vi "Generate Veristand Loopback Channels.vi"() -> (1 "Rx Aliases":string[](array[string]), 2 "Tx Aliases":string[](array[string]))   [LabVIEW 2020, in "Loopback.lvclass"]
uses:
  Loopback.lvclass
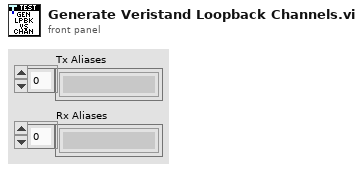
[diagram p1: front panel]
types:
  T1 = cluster{"tx terminal name":string, "rx terminal name":string, "words":i32, "parameter names":string[]}[]
  T2 = cluster{"tx terminal name":string, "rx terminal name":string, "words":i32, "parameter names":string[]}
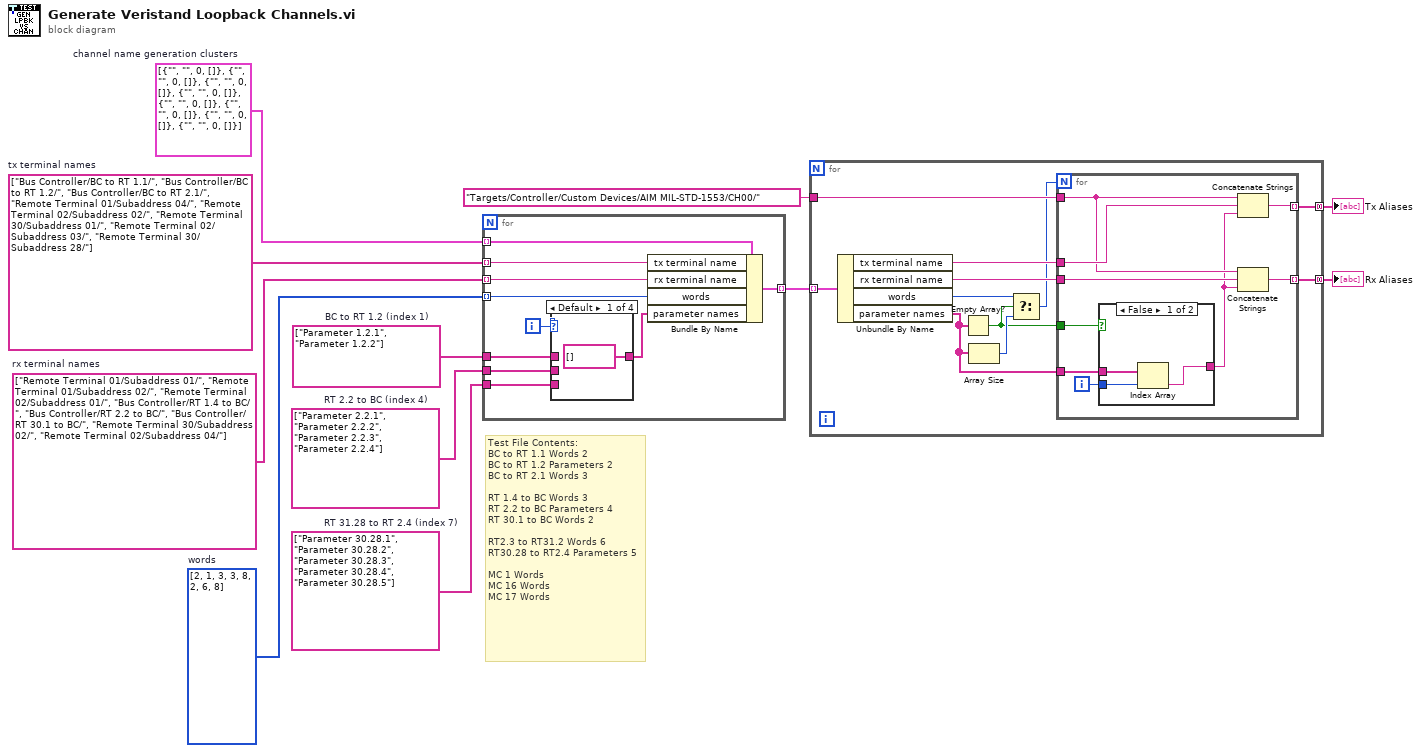
[diagram p0: block diagram]
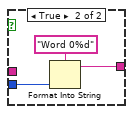
[diagram p5: hidden frame]
diagram:
  w8 = i32[] [2, 1, 3, 3, 8, 2, 6, 8]  # words
  w10 = string[] ["Remote Terminal 01/Subaddress 01/", "Remote Terminal 01/Subaddress 02/", "Remote Terminal 02/Subaddress 01/", "Bus Controller/RT 1.4 to BC/", "Bus Controller/RT 2.2 to BC/", "Bus Controller/RT 30.1 to BC/", "Remote Terminal 30/Subaddress 02/", "Remote Terminal 02/Subaddress 04/"]  # rx terminal names
  w11 = string[] ["Bus Controller/BC to RT 1.1/", "Bus Controller/BC to RT 1.2/", "Bus Controller/BC to RT 2.1/", "Remote Terminal 01/Subaddress 04/", "Remote Terminal 02/Subaddress 02/", "Remote Terminal 30/Subaddress 01/", "Remote Terminal 02/Subaddress 03/", "Remote Terminal 30/Subaddress 28/"]  # tx terminal names
  w9 = T1 [{"tx terminal name"="", "rx terminal name"="", "words"=0, "parameter names"=[]}, {"tx terminal name"="", "rx terminal name"="", "words"=0, "parameter names"=[]}, {"tx terminal name"="", "rx terminal name"="", "words"=0, "parameter names"=[]}, {"tx terminal name"="", "rx terminal name"="", "words"=0, "parameter names"=[]}, {"tx terminal name"="", "rx terminal name"="", "words"=0, "parameter names"=[]}, {"tx terminal name"="", "rx terminal name"="", "words"=0, "parameter names"=[]}, {"tx terminal name"="", "rx terminal name"="", "words"=0, "parameter names"=[]}, {"tx terminal name"="", "rx terminal name"="", "words"=0, "parameter names"=[]}]  # channel name generation clusters
  w5 = string[] ["Parameter 30.28.1", "Parameter 30.28.2", "Parameter 30.28.3", "Parameter 30.28.4", "Parameter 30.28.5"]  # RT 31.28 to RT 2.4 (index 7)
  w6 = string[] ["Parameter 2.2.1", "Parameter 2.2.2", "Parameter 2.2.3", "Parameter 2.2.4"]  # RT 2.2 to BC (index 4)
  w7 = string[] ["Parameter 1.2.1", "Parameter 1.2.2"]  # BC to RT 1.2 (index 1)
  # "Test File Contents:\nBC to RT 1.1 Words 2\nBC to RT 1.2 Parameters 2\nBC to RT 2.1 Words 3\n\nRT 1.4 to BC Words 3\nRT 2.2 to BC Parameters 4\nRT 30.1 to BC Words 2\n\nRT2.3 to RT31.2 Words 6\nRT30.28 to RT2.4 Parameters 5\n\nMC 1 Words\nMC 16 Words\nMC 17 Words"
  n1 = for {
    tunnel: w11 -> [w20] mode=indexing
    tunnel: w10 -> [w19] mode=indexing
    tunnel: w9 -> [w21] mode=indexing
    tunnel: w8 -> [w18] mode=indexing
    tunnel: w7 -> [w14]
    tunnel: w6 -> [w13]
    tunnel: w5 -> [w12]
    tunnel: [w17] -> w4 mode=indexing
    i -> [w16]
    n2 = case shown="Default" w16 {
      tunnel: [string[] [] ("parameter names") w23 w24 w25] -> w15
      tunnel: w14 -> [_ w23 _ _]
      tunnel: w13 -> [_ _ w24 _]
      tunnel: w12 -> [_ _ _ w25]
      frame Default {
      }
      frame 1 {
      }
      frame 4 {
      }
      frame 7 {
      }
    }
    n3 = Bundle By Name(cluster=w21, "tx terminal name"=w20, "rx terminal name"=w19, "words"=w18, "parameter names"=w15) -> (w17:T2)
  }
  n4 = for {
    tunnel: w4 -> [w36] mode=indexing
    tunnel: "Targets/Controller/Custom Devices/AIM MIL-STD-1553/CH00/" ("base name for channel aliases") -> [w33]
    tunnel: [w27] -> w2 mode=concatenating
    tunnel: [w26] -> w1 mode=concatenating
    n5 = Unbundle By Name(w36) -> ("tx terminal name"=w35:string, "rx terminal name"=w34:string, "words"=w31:i32, "parameter names"=w29:string[])
    n6 = Empty Array?(array=w29) -> (empty?=w28:bool)
    n7 = Array Size(array=w29) -> (size(s)=w32:i32)
    n8 = Select(t=w31, s=w28, f=w32) -> (s? t:f=w30:i32)
    n9 = for {
      N: w30 -> [_]
      tunnel: w35 -> [w45]
      tunnel: w34 -> [w44]
      tunnel: w33 -> [w43]
      tunnel: w29 -> [w39]
      tunnel: w28 -> [w42]
      tunnel: [w38] -> w27 mode=indexing
      tunnel: [w37] -> w26 mode=indexing
      i -> [w41]
      n10 = case shown="False" w42 {
        tunnel: w41 -> [w47 w51]
        tunnel: [w46 w49] -> w40
        tunnel: w39 -> [w48 _]
        frame False {
          n11 = Index Array(array=w48, index=w47) -> (element=w46:string)
        }
        frame True {
          n12 = Format Into String(format string="Word 0%d", w51) -> (resulting string=w49:string)  [unwired: 2 in, 1 out]
        }
      }
      n13 = Concatenate Strings(w43, w45, w40) -> (w37:string)
      n14 = Concatenate Strings(w43, w44, w40) -> (w38:string)
    }
  }
  "Rx Aliases" <- w2
  "Tx Aliases" <- w1
